vi "create.yearly.array.vi"(9 "end time":timestamp, 11 "start time":timestamp) -> (1 "names":string[](array[string]), 3 "timestamps":dbl[](array[numeric]))   [LabVIEW 2024]
uses:
  <vilib>/Utility/miscctls.llb/LVDateTimeRec.ctl
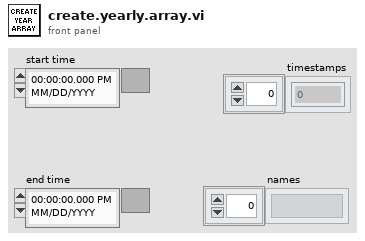
[diagram p1: front panel]
types:
  T1 = typedef "LVDateTimeRec.ctl" = cluster{"fractional second":dbl, "second":i32, "minute":i32, "hour":i32, "day of month":i32, "month":i32, "year":i32, "day of week":i32, "day of year":i32, "DST":i32}
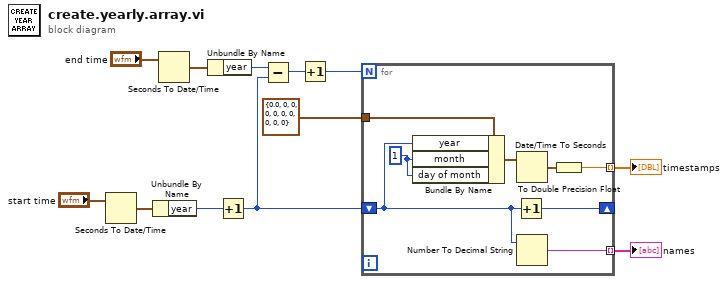
[diagram p0: block diagram]
diagram:
  n1 = Seconds To Date/Time(time stamp (now)="start time") -> (date time rec=w11:T1)  [unwired: 1 in]
  n2 = Unbundle By Name(w11) -> ("year"=w8:i32)
  n3 = Seconds To Date/Time(time stamp (now)="end time") -> (date time rec=w9:T1)  [unwired: 1 in]
  n4 = Unbundle By Name(w9) -> ("year"=w7:i32)
  n5 = Increment(x=w8) -> (x+1=w4:i32)
  n6 = Subtract(x=w7, y=w4) -> (x-y=w6:i32)
  n7 = Increment(x=w6) -> (x+1=w1:i32)
  n8 = for {
    N: w1 -> [_]
    tunnel: T1 {"fractional second"=0.0, "second"=0, "minute"=0, "hour"=0, "day of month"=0, "month"=0, "year"=0, "day of week"=0, "day of year"=0, "DST"=0} ("date time rec") -> [w20]
    shift-right: [w19] -> _
    shift-left: w4 -> [w15]
    tunnel: [w13] -> w3 mode=indexing
    tunnel: [w14] -> w2 mode=indexing
    w16 = 1 ("month")
    n9 = Bundle By Name(cluster=w20, "year"=w15, "month"=w16, "day of month"=w16) -> (w18:T1)
    n10 = Increment(x=w15) -> (x+1=w19:i32)
    n11 = Date/Time To Seconds(2:w18) -> (0:w17:timestamp)  [unwired: 1 in]
    n12 = Number To Decimal String(number=w15) -> (decimal integer string=w14:string)  [unwired: 1 in]
    n13 = To Double Precision Float(number=w17) -> (double precision float=w13:dbl)
  }
  "timestamps" <- w3
  "names" <- w2
